vi "Y_profile_sawtooth.vi"(1 "Vy min(bits)":i16, 3 "line counter":u16, 6 "y step size":u16) -> (0 "y signal":i16)   [LabVIEW 2010]
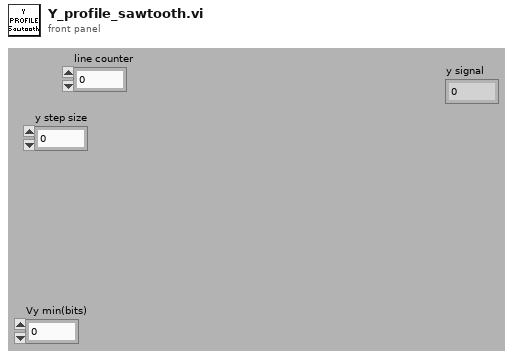
[diagram p1: front panel]
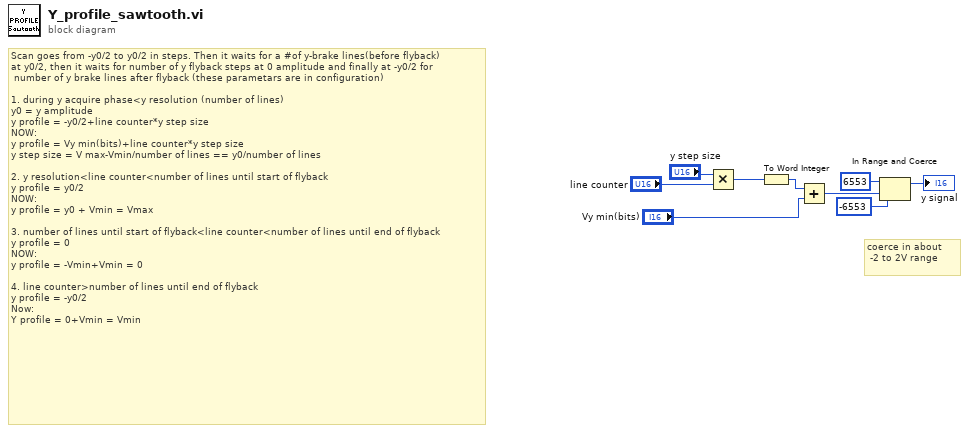
[diagram p0: block diagram]
diagram:
  # "coerce in about\n -2 to 2V range"
  # "Scan goes from -y0/2 to y0/2 in steps. Then it waits for a #of y-brake lines(before flyback) \nat y0/2, then it waits for number of y flyback steps at 0 amplitude and finally at -y0/2 for\n number of y brake lines after flyback (these parametars are in configuration)\n\n1. during y acquire phase<y resolution (number of lines)\ny0 = y amplitude\ny profile = -y0/2+line counter*y step size\nNOW:\ny profile = Vy min(bits)+line counter*y step size\ny step size = V max-Vmin/number of lines == y0/number of lines\n\n2. y resolution<line counter<number of lines until start of flyback\ny profile = y0/2\nNOW:\ny profile = y0 + Vmin = Vmax\n\n3. number of lines until start of flyback<line counter<number of lines until end of flyback\ny profile = 0\nNOW:\ny profile = -Vmin+Vmin = 0\n\n4. line counter>number of lines until end of flyback\ny profile = -y0/2\nNow:\nY profile = 0+Vmin = Vmin"
  n1 = Multiply(x="y step size", y="line counter") -> (x*y=w1:u16)
  n2 = To Word Integer(number=w1) -> (16bit integer=w7:i16)
  n3 = Add(x=w7, y="Vy min(bits)") -> (x+y=w5:i16)
  n4 = In Range and Coerce(upper limit=i16 6553, x=w5, lower limit=i16 -6553) -> (coerced(x)=→"y signal":i16)  [unwired: 1 out]
